vi "Add Block Diagram Content.vi"(8 "error in (no error)":errorcluster, 9 "Term Refnums":refnum<vi>[](array[refnum]), 10 "ModuleLoop":T1, 11 "FPGA Addon Input.lvclass":refnum<class "FPGA Addon Input.lvclass">) -> (0 "error out":errorcluster, 3 "FPGA Addon Input.lvclass":refnum<class "FPGA Addon Input.lvclass">)   [LabVIEW 2025, in "FPGA Addon Input.lvclass"]
uses:
  FPGA Addon Input.lvclass
  VI/VI/Module.Refs.ctl
  <vilib>/Utility/miscctls.llb/LVPointTypeDef.ctl
  <vilib>/_script/New VI Object TypeDefs/NewVIObject_LVRelativePositionTypeDef.ctl
  <vilib>/_script/New VI Object TypeDefs/NewVIObject_LVRelativeDirectionTypeDef.ctl
  <vilib>/Utility/miscctls.llb/LVPoint32TypeDef.ctl
  Signal/Read IP Core Path.vi
  Signal/Read Signal Name.vi
  VI/VI/VI.lvclass
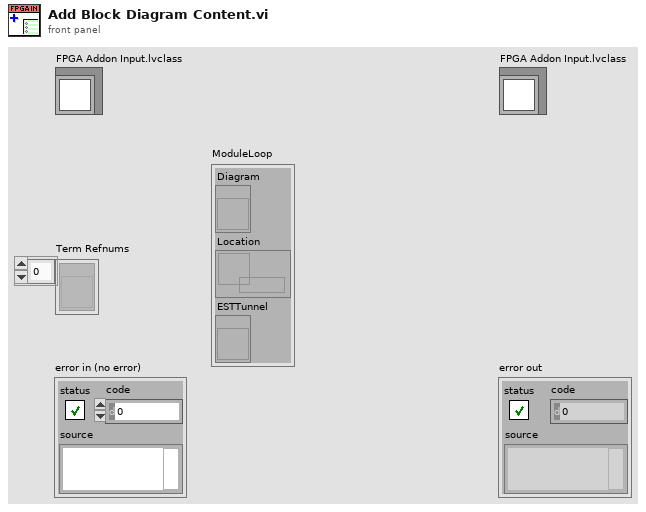
[diagram p1: front panel]
types:
  T1 = typedef "VI.lvclass/Module.Refs.ctl" = cluster{"Diagram":refnum<vi>, "Location":refnum<data-value>, "ESTTunnel":refnum<vi>}
  T2 = typedef "NewVIObject_LVRelativePositionTypeDef.ctl" = cluster{"Refnum":refnum<vi>, "Relative Direction":T3, "Point32":T4}
  T3 = typedef "NewVIObject_LVRelativeDirectionTypeDef.ctl" = enum32{"Right", "Left", "Top", "Bottom", "Top Right", "Top Left", "Bottom Right", "Bottom Left"}
  T4 = typedef "LVPoint32TypeDef.ctl" = cluster{"Horizontal":i32, "Vertical":i32}
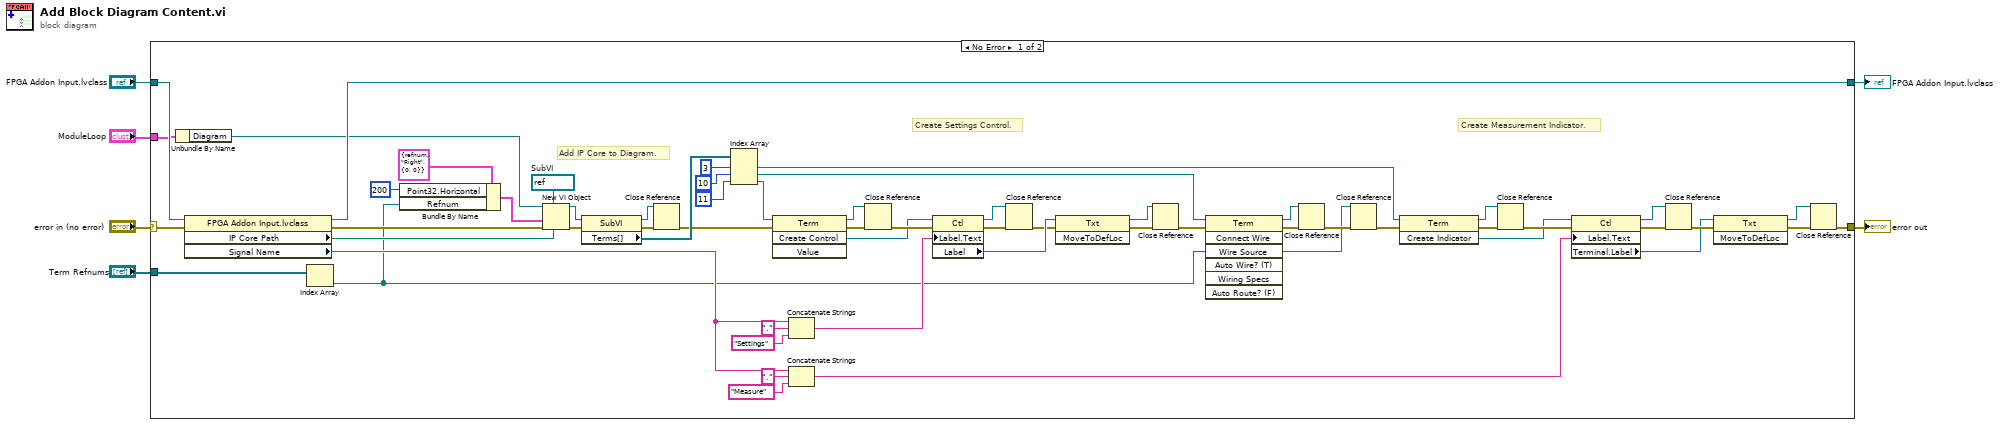
[diagram p0: block diagram]
diagram:
  n1 = case shown="No Error" "error in (no error)" {
    selector: "error in (no error)" -> [w11 w65]
    tunnel: "FPGA Addon Input.lvclass" -> [w64 w66]
    tunnel: [w63 w66] -> w5
    tunnel: "ModuleLoop" -> [w62 _]
    tunnel: [w16 w65] -> w3
    tunnel: "Term Refnums" -> [w15 _]
    frame No Error {
      w33 = refnum<vi> refnum  # SubVI
      # "Create Measurement Indicator."
      # "Create Settings Control."
      # "Add IP Core to Diagram."
      n2 = Unbundle By Name(w62) -> ("Diagram"=w14:refnum<vi>)
      n3 = property class="FPGA Addon Input.lvclass"(reference=w64, error in=w11) -> (reference out=w63:refnum<class "FPGA Addon Input.lvclass">, error out=w17:errorcluster, "IP Core Path"=w13:path, "Signal Name"=w12:string)
      n4 = Index Array(array=w15) -> (element=w7:refnum<vi>)  [unwired: 1 in]
      n5 = Bundle By Name(cluster=T2 {"Refnum"=refnum, "Relative Direction"=enum."Right", "Point32"={"Horizontal"=0, "Vertical"=0}} ("Relative Position"), "Point32.Horizontal"=200, "Refnum"=w7) -> (w18:T2)
      n6 = New VI Object(vi object class=w33, owner refnum=w14, position/next to=w18, 6:w13, 8:w17) -> (object refnum=w37:refnum<vi>, 0:w38:errorcluster)  [unwired: 3 in]
      n7 = property class="SubVI"(reference=w37, error in=w38) -> (reference out=w9:refnum<vi>, error out=w10:errorcluster, "Terms[]"=w34:refnum<vi>[])
      n8 = Close Reference(reference=w9, error in (no error)=w10) -> (error out=w8:errorcluster)
      n9 = Index Array(array=w34, index #1=3 ("index"), index #2=10 ("index"), index #3=11 ("index")) -> (element #1=w51:refnum<vi>, element #2=w42:refnum<vi>, element #3=w52:refnum<vi>)
      n10 = invoke class="Term" method="Create Control"(reference=w52, error in=w8) -> (reference out=w49:refnum<vi>, error out=w48:errorcluster, "Create Control"=w32:refnum<vi>)  [unwired: 2 in, 1 out]
      n11 = Concatenate Strings(w12, "." ("string"), "Settings" ("string")) -> (w39:string)
      n12 = Concatenate Strings(w12, "." ("string"), "Measure" ("string")) -> (w47:string)
      n13 = Close Reference(reference=w49, error in (no error)=w48) -> (error out=w50:errorcluster)
      n14 = property class="Ctl"(reference=w32, error in=w50, "Label.Text"=w39) -> (reference out=w31:refnum<vi>, error out=w29:errorcluster, "Label"=w30:refnum<vi>)
      n15 = Close Reference(reference=w31, error in (no error)=w29) -> (error out=w28:errorcluster)
      n16 = invoke class="Txt" method="MoveToDefLoc"(reference=w30, error in=w28) -> (reference out=w26:refnum<vi>, error out=w27:errorcluster)  [unwired: 1 in, 1 out]
      n17 = Close Reference(reference=w26, error in (no error)=w27) -> (error out=w25:errorcluster)
      n18 = invoke class="Term" method="Connect Wire"(reference=w42, error in=w25, "Wire Source"=w7) -> (reference out=w54:refnum<vi>, error out=w53:errorcluster)  [unwired: 4 in, 5 out]
      n19 = Close Reference(reference=w54, error in (no error)=w53) -> (error out=w55:errorcluster)
      n20 = Close Reference(reference=w7, error in (no error)=w55) -> (error out=w56:errorcluster)
      n21 = invoke class="Term" method="Create Indicator"(reference=w51, error in=w56) -> (reference out=w59:refnum<vi>, error out=w60:errorcluster, "Create Indicator"=w44:refnum<vi>)  [unwired: 1 in]
      n22 = Close Reference(reference=w59, error in (no error)=w60) -> (error out=w61:errorcluster)
      n23 = property class="Ctl"(reference=w44, error in=w61, "Label.Text"=w47) -> (reference out=w57:refnum<vi>, error out=w58:errorcluster, "Terminal.Label"=w22:refnum<vi>)
      n24 = Close Reference(reference=w57, error in (no error)=w58) -> (error out=w23:errorcluster)
      n25 = invoke class="Txt" method="MoveToDefLoc"(reference=w22, error in=w23) -> (reference out=w21:refnum<vi>, error out=w24:errorcluster)  [unwired: 1 in, 1 out]
      n26 = Close Reference(reference=w21, error in (no error)=w24) -> (error out=w16:errorcluster)
    }
    frame Error {
    }
  }
  "error out" <- w3
  "FPGA Addon Input.lvclass" <- w5
